vi "exit_event.get.vi"(11 "librarian_sm in":refnum<class "librarian.lvclass">) -> (2 "exit event":refnum<user-event>, 3 "librarian_sm out":refnum<class "librarian.lvclass">)   [LabVIEW 2020, in "librarian.lvclass"]
uses:
  librarian.lvclass
  librarian.lvclass/librarian.ctl
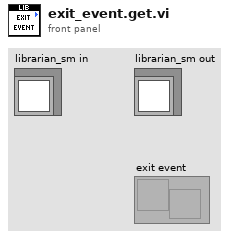
[diagram p1: front panel]
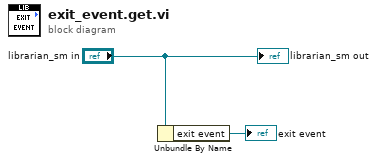
[diagram p0: block diagram]
diagram:
  n1 = Unbundle By Name("librarian_sm in") -> ("exit event"=→"exit event":refnum<user-event>)
  "librarian_sm out" <- "librarian_sm in"
